vi "ARGBExtractChannel.vi"(7 "ExtractOperation":T1, 8 "error in (no error)":errorcluster, 10 "Greyscale Image Destination":T2, 11 "ARGB Image Source":T3) -> (0 "error out":errorcluster)   [LabVIEW 2020, in "image.lvlib"]
uses:
  image.lvlib
  ARGB Image.ctl
  Greyscale Image.ctl
  ExtractOptions.ctl
  common/common.lvlib
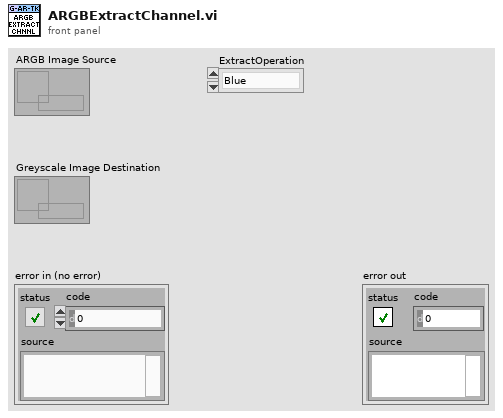
[diagram p1: front panel]
types:
  T1 = typedef "image.lvlib/ExtractOptions.ctl" = enum8{"Blue", "Green", "Red", "Alpha", "Greyscale"}
  T2 = typedef "image.lvlib/Greyscale Image.ctl" = refnum<data-value>
  T3 = typedef "image.lvlib/ARGB Image.ctl" = refnum<data-value>
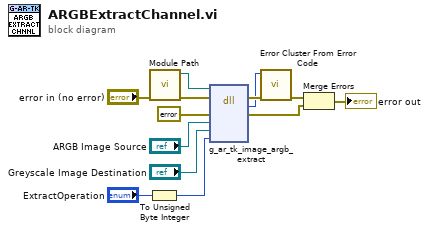
[diagram p0: block diagram]
diagram:
  n1 = To Unsigned Byte Integer(number="ExtractOperation") -> (unsigned 8bit integer=w3:u8)
  n2 = call "Module Path.vi"("error in (no error)"="error in (no error)") -> ("error out"=w2:errorcluster, "Path"=w1:path)  [unwired: 9 in]
  n3 = dll-call lib="?" fn="g_ar_tk_image_argb_extract"(path in=w1, error in=w2, "error_cluster"=errorcluster {"status"=FALSE, "code"=0, "source"=""} ("error constant"), "EDVR src"="ARGB Image Source", "EDVR dst"="Greyscale Image Destination", "operation"=w3) -> (error out=w13:errorcluster, "MgErr"=w12:i32, "error_cluster"=w9:errorcluster)  [unwired: 4 in, 1 out]
  n4 = call <vilib>:"Error Cluster From Error Code.vi"("error in (no error)"=w13, "error code (0)"=w12) -> ("error out"=w11:errorcluster)  [unwired: 7 in]
  n5 = Merge Errors(w11, w9) -> (→"error out":errorcluster)
